vi "GOMDBTS2048 get Serial Number.vi"(8 "error in (no error)":errorcluster, 11 "handle":i32) -> (0 "error out":errorcluster, 2 "function return":i32, 3 "value":string)   [LabVIEW 2015, in "GOMDBTS2048.lvlib"]
doc: "GOBTS2048DLL int __stdcall GOMDBTS2048_getDLLVersion(char* value);"
uses:
  GOMDBTS2048.lvlib
  runtime/GOMDBTS2048.dll
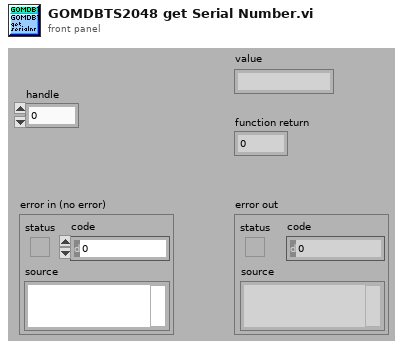
[diagram p1: front panel]
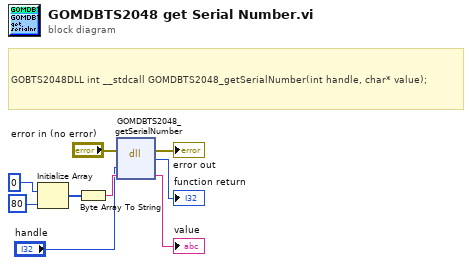
[diagram p0: block diagram]
diagram:
  # "GOBTS2048DLL int __stdcall GOMDBTS2048_getSerialNumber(int handle, char* value);"
  n1 = Initialize Array(u8 0 ("element"), 80 ("dimension size")) -> (w8:u8[])
  n2 = Byte Array To String(unsigned byte array=w8) -> (string=w7:string)
  n3 = dll-call lib="C:/Users/rkoch/Documents/GO_Library/runtime/GOMDBTS2048.*" fn="GOMDBTS2048_getSerialNumber"(error in="error in (no error)", "handle"="handle", "value"=w7) -> (error out=→"error out":errorcluster, "return type"=→"function return":i32, "value"=→"value":string)  [unwired: 3 in, 1 out]
